vi "IETemplateVIFolderConstant.vi"() -> (15 "IE VI templates":path)   [LabVIEW 2021]
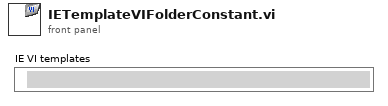
[diagram p1: front panel]
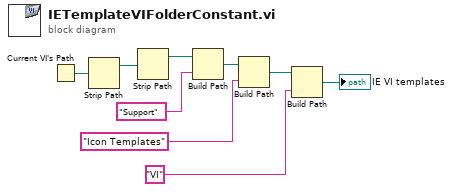
[diagram p0: block diagram]
diagram:
  n1 = Current VI's Path() -> (path=w9:path)
  n2 = Strip Path(path=w9) -> (stripped path=w8:path)  [unwired: 1 out]
  n3 = Strip Path(path=w8) -> (stripped path=w7:path)  [unwired: 1 out]
  n4 = Build Path(base path=w7, name or relative path="Support") -> (appended path=w5:path)
  n5 = Build Path(base path=w5, name or relative path="Icon Templates") -> (appended path=w3:path)
  n6 = Build Path(base path=w3, name or relative path="VI") -> (appended path=→"IE VI templates":path)
